vi "Riccati_DARE.vi"(8 "R":T1, 9 "Q":T1, 10 "B":T1, 11 "A":T1) -> (0 "error out":errorcluster, 1 "Error":bool, 2 "Iterations":i32, 3 "Answer":T1)   [LabVIEW 2019, in "Trajectory_Library.lvlib"]
doc: "Solves the discrete alegebraic Riccati equation.\n \nInput:\n - A -- System matrix.\n - B -- nput matrix.\n - Q -- State cost matrix.\n - R -- Input cost matrix.\n\nOutputs:\n Answer -- Solution of DARE.\n iterations -- Number of iterations\n error -- If TRUE, an error occured"
uses:
  Trajectory_Library.lvlib
  <vilib>/Analysis/Matrix/Datatypes/RealMatrix.ctl
  <vilib>/Analysis/Matrix/NI_Matrix.lvlib
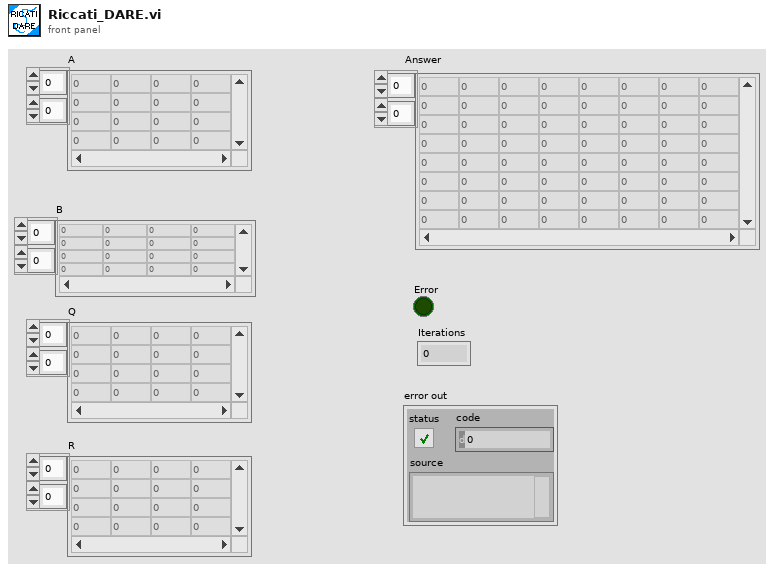
[diagram p1: front panel]
types:
  T1 = typedef "NI_Matrix.lvlib/RealMatrix.ctl" = dbl[][]
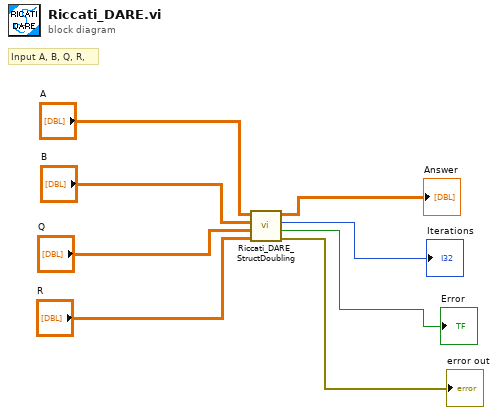
[diagram p0: block diagram]
diagram:
  # "Input A, B, Q, R,"
  n1 = call "Riccati_DARE_StructDoubling.vi"("R"="R", "Q"="Q", "B"="B", "A"="A") -> ("error out"=→"error out":errorcluster, "Error"=→"Error":bool, "Iterations"=→"Iterations":i32, "Answer"=→"Answer":T1)  [unwired: 4 in]
